vi "76_Vision_RC Servo_DC_Moto_4.vi"() -> ()   [LabVIEW 2018]
uses:
  <userlib>/KNR OS 4.0 LabVIEW Toolkit/Type Definition/Resource.ctl
  <userlib>/KNR OS 4.0 LabVIEW Toolkit/Type Definition/RC Servo Port.ctl
  <userlib>/KNR OS 4.0 LabVIEW Toolkit/Type Definition/DC Motor Port.ctl
panel:
  out "area":dbl
  out "RC Pulse Width (uS)":u16[](array[numeric])
  out "Image Out":T1(plugin-control)
  in  "stop":bool
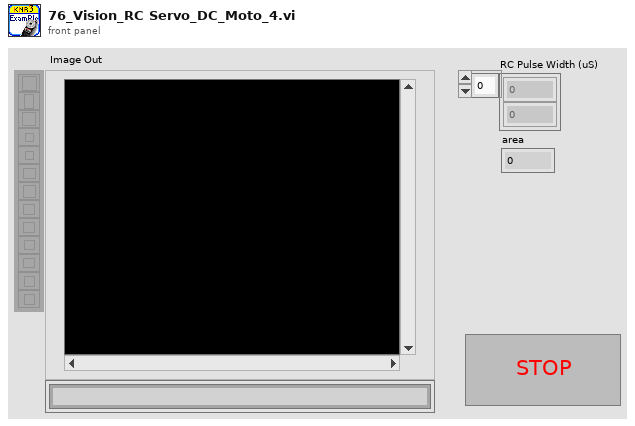
[diagram p1: front panel]
types:
  T1 = typedef "IMAQ Image.ctl" = refnum<image>
  T2 = typedef "DC Motor Port.ctl" = u16
  T3 = typedef "RC Servo Port.ctl" = u16
  T4 = typedef "Resource.ctl" = enum16{"KNRm_DDRC", "KNRm_DDDD", "KNRm_DDDR", "KNRm_DDDC", "KNR", "KNRm_neww"}
  T5 = typedef "KNR3 Reference.ctl" = cluster{"FPGA Session":refnum<class "FPGA Interface Base.lvclass">, "Resource":T4}
  T6 = cluster{"Left":dbl, "Top":dbl, "Right":dbl, "Bottom":dbl}
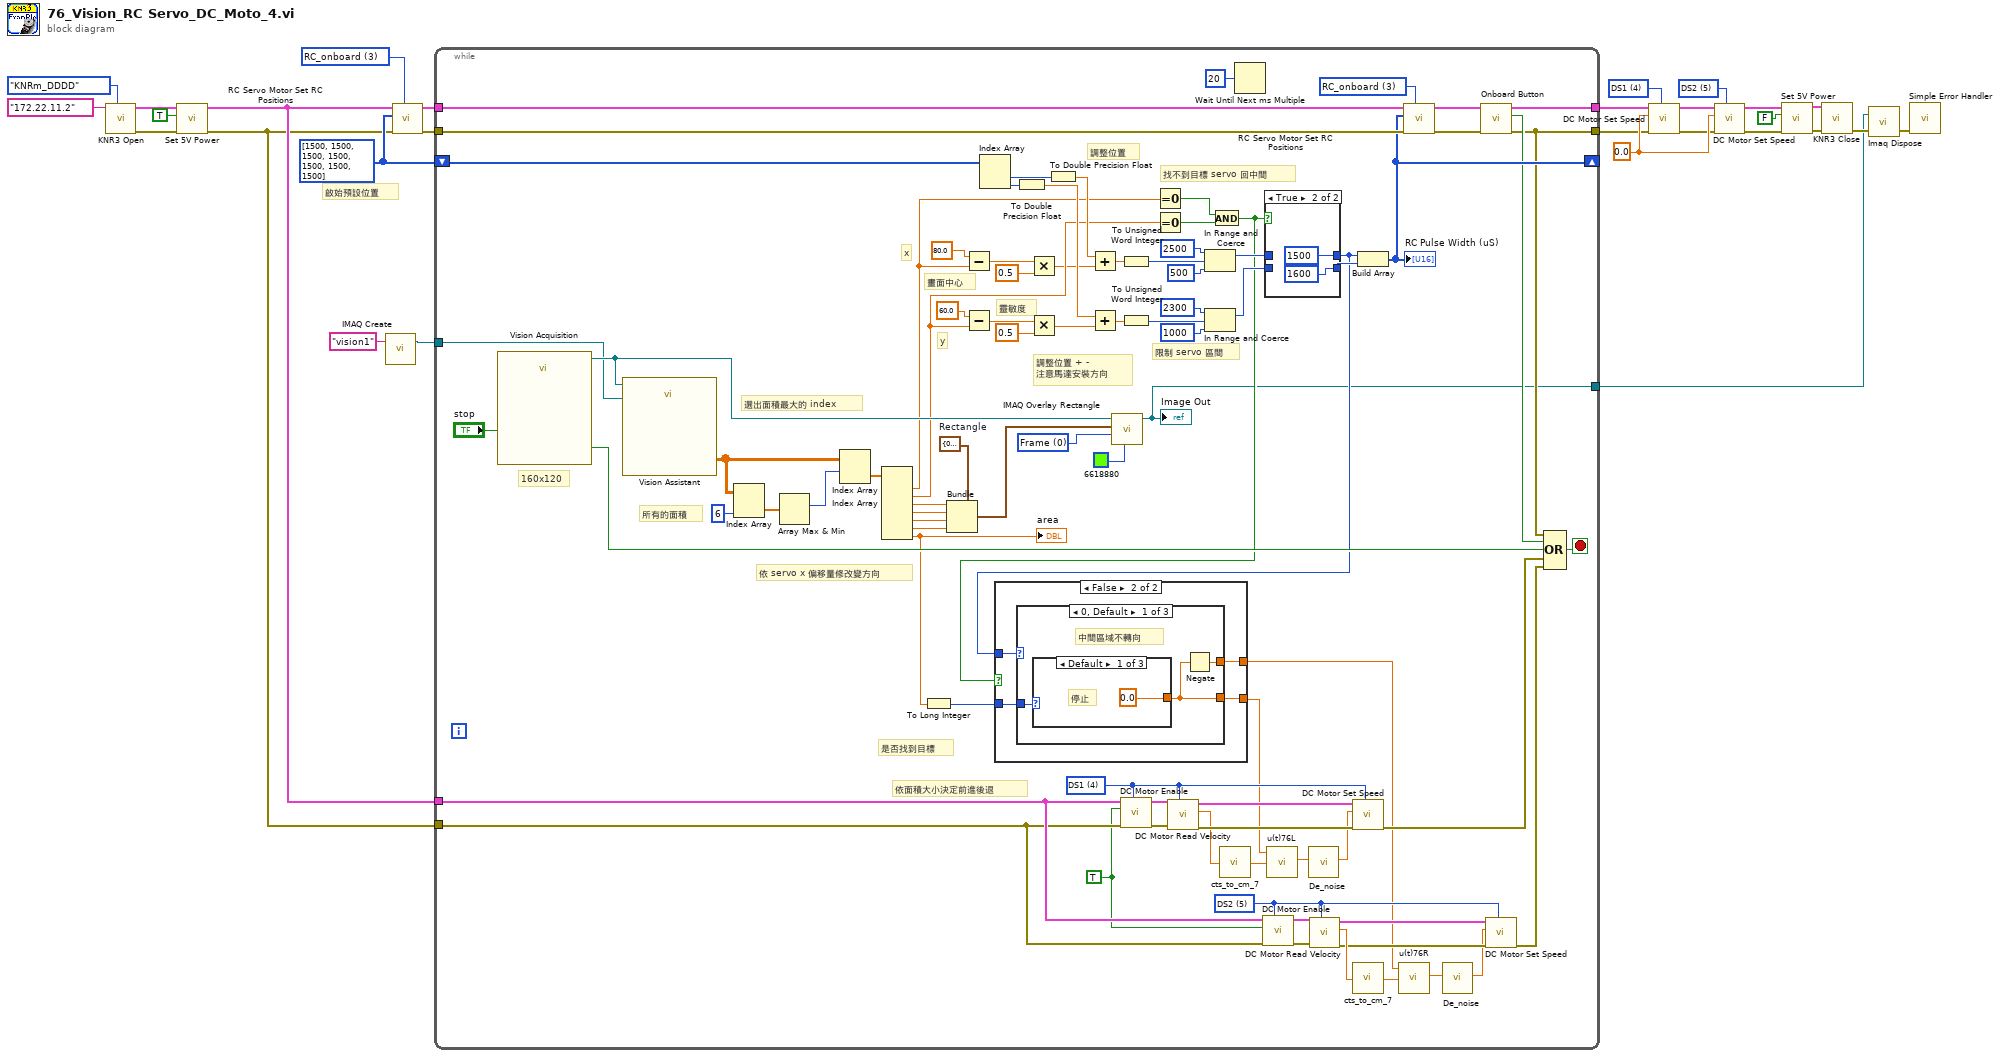
[diagram p0: block diagram]
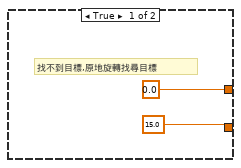
[diagram p2: hidden frame]
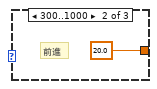
[diagram p3: hidden frame]
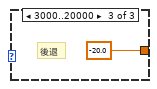
[diagram p4: hidden frame]
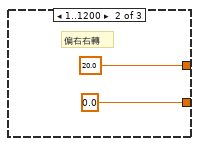
[diagram p5: hidden frame]
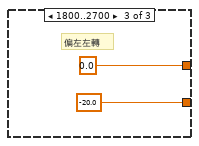
[diagram p6: hidden frame]
diagram:
  w7 = T2 5 items=["DS1"=4, "DS2"=5, "DS3"=6, "DS4"=7] ("Port (DS1)")
  w8 = T2 4 items=["DS1"=4, "DS2"=5, "DS3"=6, "DS4"=7] ("Port (DS1)")
  w9 = 0.0 ("Speed (+-100%)")
  w18 = u16[] [1500, 1500, 1500, 1500, 1500, 1500, 1500] ("RC Pulse Width (1500 uS)")
  w21 = T3 3 items=["RC_onboard"=3, "RC_box"=9] ("Port (RC_onboard)")
  # "啟始預設位置"
  n1 = call <userlib>:"KNR3 Open.vi"("Resource"=Resource."KNRm_DDDD", "IP"="172.22.11.2") -> ("error out"=w26:errorcluster, "KNR out"=w27:T5)  [unwired: 8 in]
  n2 = call <userlib>:"Set 5V Power.vi"("error in (no error)"=w26, "5V Power(T)"=TRUE ("5V Power"), "KNR in"=w27) -> ("error out"=w16:errorcluster, "KNR out"=w17:T5)  [unwired: 7 in]
  n3 = call "IMAQ Create"("Image Name"="vision1") -> ("New Image"=w19:T1)  [unwired: 4 in, 1 out]
  n4 = call <userlib>:"RC Servo Motor Set RC Positions.vi"("Port (RC_onboard)"=w21, "RC Pulse Width (1500 uS)"=w18, "KNR in"=w17) -> ("KNR out"=w22:T5)  [unwired: 7 in, 1 out]
  n5 = while {
    tunnel: w22 -> [w112]
    tunnel: [w43] -> w15
    tunnel: w16 -> [w110]
    tunnel: [w41] -> w6
    tunnel: w19 -> [w93]
    shift-right: [w77] -> _
    shift-left: w18 -> [w80]
    tunnel: w17 -> [w47]
    tunnel: w16 -> [w46]
    tunnel: [w33] -> w1
    stop <- w109 stop-if-true
    w45 = u32 0 items=["Frame", "Fill", "Highlight"] ("Drawing Mode (Frame)")
    w49 = T2 5 items=["DS1"=4, "DS2"=5, "DS3"=6, "DS4"=7] ("Port 2")
    w44 = TRUE ("Enable Motor(F)")
    w61 = T2 4 items=["DS1"=4, "DS2"=5, "DS3"=6, "DS4"=7] ("Port 2")
    w105 = T6 {"Left"=0.0, "Top"=0.0, "Right"=0.0, "Bottom"=0.0}  # Rectangle
    w107 = T3 3 items=["RC_onboard"=3, "RC_box"=9] ("RC Motor")
    # "依面積大小決定前進後退"
    # "依 servo x 偏移量修改變方向"
    # "是否找到目標"
    # "調整位置 + -\n注意馬達安裝方向"
    # "調整位置"
    # "靈敏度"
    # "所有的面積"
    # "畫面中心"
    # "限制 servo 區間"
    # "找不到目標 servo 回中間"
    # "y"
    # "x"
    # "160x120"
    # "選出面積最大的 index"
    n6 = call "Vision Acquisition"("Stop (F)"="stop") -> ("Image Out"=w98:T1, "Stopped"=w91:bool)  [unwired: 24 in, 1 out]
    n7 = call "Vision Assistant"("Image In"=w98, "Image Dst"=w93) -> ("Particle Measurements (Pixels) (Particle Analysis 1)"=w97:dbl[][])  [unwired: 22 in, 3 out]
    n8 = Index Array "Index Array"(array=w97, index (col)=6 ("disabled index (col)")) -> (element=w96:dbl[])  [unwired: 1 in]
    n9 = Array Max & Min(array=w96) -> (max index (indices)=w95:i32)  [unwired: 3 out]
    n10 = Index Array "Index Array"(array=w97, index (row)=w95) -> (element=w106:dbl[])  [unwired: 1 in]
    n11 = Index Array "Index Array"(array=w106) -> (element #1=w70:dbl, element #2=w69:dbl, element #3=w104:dbl, element #4=w103:dbl, element #5=w102:dbl, element #6=w101:dbl, element #7=w55:dbl)  [unwired: 7 in]
    "area" <- w55
    n12 = To Long Integer(number=w55) -> (32bit integer=w36:i32)
    n13 = Bundle "Bundle"(cluster=w105, "Left"=w104, "Top"=w103, "Right"=w102, "Bottom"=w101) -> (w100:T6)
    n14 = Subtract(x=80.0 ("y"), y=w70) -> (x-y=w87:dbl)
    n15 = Subtract(x=60.0 ("y"), y=w69) -> (x-y=w88:dbl)
    n16 = Index Array "Index Array"(array=w80) -> (element #1=w79:u16, element #2=w78:u16)  [unwired: 2 in]
    n17 = To Double Precision Float(number=w78) -> (double precision float=w71:dbl)
    n18 = Multiply(x=w87, y=0.5) -> (x*y=w68:dbl)
    n19 = Multiply(x=w88, y=0.5) -> (x*y=w67:dbl)
    n20 = To Double Precision Float(number=w79) -> (double precision float=w72:dbl)
    n21 = Add(x=w72, y=w68) -> (x+y=w89:dbl)
    n22 = Add(x=w71, y=w67) -> (x+y=w90:dbl)
    n23 = call "IMAQ Overlay Rectangle"("Color"=u32 6618880, "Drawing Mode (Frame)"=w45, "Rectangle"=w100, "Image"=w98) -> ("Image Out"=w33:T1)  [unwired: 6 in, 1 out]
    "Image Out" <- w33
    n24 = To Unsigned Word Integer(number=w89) -> (unsigned 16bit integer=w74:u16)
    n25 = To Unsigned Word Integer(number=w90) -> (unsigned 16bit integer=w73:u16)
    n26 = call <userlib>:"DC Motor Enable.vi"("Port (DS1)"=w61, "error in (no error)"=w46, "Enable Motor(F)"=w44, "KNR in"=w47) -> ("error out"=w57:errorcluster, "KNR out"=w56:T5)  [unwired: 6 in]
    n27 = Equal To 0?(x=w70) -> (x = 0?=w65:bool)
    n28 = Equal To 0?(x=w69) -> (x = 0?=w66:bool)
    n29 = call <userlib>:"DC Motor Read Velocity.vi"("Port (DS1)"=w61, "error in (no error)"=w57, "KNR in"=w56) -> ("error out"=w60:errorcluster, "Velocity (cts/sec)"=w58:dbl, "KNR out"=w59:T5)  [unwired: 6 in]
    n30 = In Range and Coerce(upper limit=u16 2500, x=w74, lower limit=u16 500) -> (coerced(x)=w64:u16)  [unwired: 1 out]
    n31 = In Range and Coerce(upper limit=u16 2300, x=w73, lower limit=u16 1000) -> (coerced(x)=w63:u16)  [unwired: 1 out]
    n32 = And(x=w65, y=w66) -> (x .and. y?=w34:bool)
    n33 = call "cts_to_cm_7.vi"("cts"=w58) -> ("cm"=w31:dbl)
    n34 = Wait Until Next ms Multiple(millisecond multiple=u32 20) -> ()  [unwired: 1 out]
    n35 = call <userlib>:"DC Motor Enable.vi"("Port (DS1)"=w49, "error in (no error)"=w46, "Enable Motor(F)"=w44, "KNR in"=w47) -> ("error out"=w53:errorcluster, "KNR out"=w54:T5)  [unwired: 6 in]
    n36 = case shown="True" w34 {
      tunnel: w64 -> [w130 _]
      tunnel: w63 -> [w129 _]
      tunnel: [w130 u16 1500] -> w37
      tunnel: [w129 u16 1600] -> w62
      frame False {
      }
      frame True {
      }
    }
    n37 = case shown="False" w34 {
      tunnel: w37 -> [_ w118]
      tunnel: w36 -> [_ w117]
      tunnel: [15.0 w116] -> w32
      tunnel: [0.0 w115] -> w30
      frame True {
        # "找不到目標,原地旋轉找尋目標"
      }
      frame False {
        n38 = case shown="0, Default" w118 {
          tunnel: [w120 0.0 -20.0] -> w116
          tunnel: [w121 20.0 0.0] -> w115
          tunnel: w117 -> [w119 _ _]
          frame 0, Default {
            # "中間區域不轉向"
            n39 = case shown="Default" w119 {
              tunnel: [0.0 20.0 -20.0] -> w120
              frame Default {
                # "停止"
              }
              frame 300..1000 {
                # "前進"
              }
              frame 3000..20000 {
                # "後退"
              }
            }
            n40 = Negate(x=w120) -> (-x=w121:dbl)
          }
          frame 1..1200 {
            # "偏右右轉"
          }
          frame 1800..2700 {
            # "偏左左轉"
          }
        }
      }
    }
    n41 = call "u(t)76L.vi"("Velocity"=w31, "Desire Velosity"=w32) -> ("u(t)"=w39:dbl)  [unwired: 6 in]
    n42 = call "De_noise.vi"("u(t)"=w39) -> ("u(t)2"=w40:dbl)  [unwired: 6 in]
    n43 = call <userlib>:"DC Motor Read Velocity.vi"("Port (DS1)"=w49, "error in (no error)"=w53, "KNR in"=w54) -> ("error out"=w50:errorcluster, "Velocity (cts/sec)"=w52:dbl, "KNR out"=w51:T5)  [unwired: 6 in]
    n44 = call <userlib>:"DC Motor Set Speed.vi"("Port (DS1)"=w61, "error in (no error)"=w60, "Speed (+-100%)"=w40, "KNR in"=w59) -> ("error out"=w35:errorcluster)  [unwired: 6 in, 1 out]
    n45 = call "cts_to_cm_7.vi"("cts"=w52) -> ("cm"=w29:dbl)
    n46 = Build Array "Build Array"(w37, w62) -> (w77:u16[])
    "RC Pulse Width (uS)" <- w77
    n47 = call "u(t)76R.vi"("Desire Velosity"=w30, "Velocity"=w29) -> ("u(t)"=w28:dbl)  [unwired: 5 in]
    n48 = call <userlib>:"RC Servo Motor Set RC Positions.vi"("Port (RC_onboard)"=w107, "error in (no error)"=w110, "RC Pulse Width (1500 uS)"=w77, "KNR in"=w112) -> ("error out"=w41:errorcluster, "KNR out"=w111:T5)  [unwired: 6 in]
    n49 = call "De_noise.vi"("u(t)"=w28) -> ("u(t)2"=w38:dbl)  [unwired: 6 in]
    n50 = call <userlib>:"Onboard Button.vi"("KNR in"=w111) -> ("value"=w42:bool, "KNR out"=w43:T5)  [unwired: 8 in, 1 out]
    n51 = call <userlib>:"DC Motor Set Speed.vi"("Port (DS1)"=w49, "error in (no error)"=w50, "Speed (+-100%)"=w38, "KNR in"=w51) -> ("error out"=w48:errorcluster)  [unwired: 6 in, 1 out]
    n52 = Compound Arithmetic op=OR(w41, w42, w91, w35, w48) -> (w109:bool)
  }
  n53 = call <userlib>:"DC Motor Set Speed.vi"("Port (DS1)"=w8, "error in (no error)"=w6, "Speed (+-100%)"=w9, "KNR in"=w15) -> ("error out"=w5:errorcluster, "KNR out"=w11:T5)  [unwired: 6 in]
  n54 = call <userlib>:"DC Motor Set Speed.vi"("Port (DS1)"=w7, "error in (no error)"=w5, "Speed (+-100%)"=w9, "KNR in"=w11) -> ("error out"=w4:errorcluster, "KNR out"=w10:T5)  [unwired: 6 in]
  n55 = call <userlib>:"Set 5V Power.vi"("error in (no error)"=w4, "5V Power(T)"=FALSE, "KNR in"=w10) -> ("error out"=w13:errorcluster, "KNR out"=w14:T5)  [unwired: 7 in]
  n56 = call <userlib>:"KNR3 Close.vi"("error in (no error)"=w13, "KNR in"=w14) -> ("error out"=w3:errorcluster)  [unwired: 9 in]
  n57 = call "Imaq Dispose"("Image"=w1, "error in (no error)"=w3) -> ("error out"=w2:errorcluster)  [unwired: 4 in]
  n58 = call <vilib>:"Simple Error Handler.vi"("error in (no error)"=w2) -> ()  [unwired: 4 in, 5 out]
